vi "MAXI GAUGE - TREE.vi"   [LabVIEW 2013, in "Maxi Gauge.lvlib"]
uses:
  <instrlib>/Maxi Gauge/Maxi Gauge.lvlib
panel:
  # "SEE DIAGRAM FOR VI TREE"
  # "Pfeiffer Vacuum GmbH\n Berlinerstrasse 43\n D-35614 Asslar\n\n Telefon +49-6441/802-0\n Telefax +49-6441/802-202\n Internet: http://www.pfeiffer-vacuum.de"
  # "Maxi Gauge"
  # "07.01.2001 FPF"
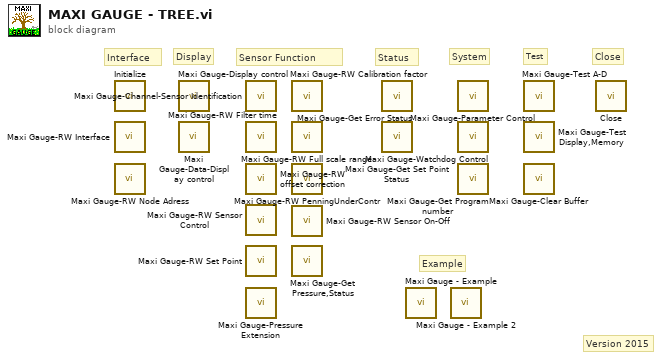
[diagram p0: block diagram]
diagram:
  # "Example"
  # "Close"
  # "Version 2015"
  # "Test"
  # "System"
  # "Status"
  # "Sensor Function"
  # "Display"
  # "Interface"
  n1 = call <instrlib>:"Initialize.vi"() -> ()  [unwired: 10 in, 2 out]
  n2 = call <instrlib>:"Maxi Gauge-RW Interface.vi"() -> ()  [unwired: 9 in, 3 out]
  n3 = call <instrlib>:"Maxi Gauge-RW Node Adress.vi"() -> ()  [unwired: 9 in, 3 out]
  n4 = call <instrlib>:"Maxi Gauge-Display control.vi"() -> ()  [unwired: 12 in, 4 out]
  n5 = call <instrlib>:"Maxi Gauge-Data-Display control.vi"() -> ()  [unwired: 11 in, 5 out]
  n6 = call <instrlib>:"Maxi Gauge-Channel-Sensor Identification.vi"() -> ()  [unwired: 8 in, 4 out]
  n7 = call <instrlib>:"Maxi Gauge-RW Filter time.vi"() -> ()  [unwired: 12 in, 8 out]
  n8 = call <instrlib>:"Maxi Gauge-RW offset correction.vi"() -> ()  [unwired: 12 in, 8 out]
  n9 = call <instrlib>:"Maxi Gauge-RW Sensor Control.vi"() -> ()  [unwired: 14 in, 6 out]
  n10 = call <instrlib>:"Maxi Gauge-RW Set Point.vi"() -> ()  [unwired: 11 in, 5 out]
  n11 = call <instrlib>:"Maxi Gauge-Pressure Extension.vi"() -> ()  [unwired: 12 in, 8 out]
  n12 = call <instrlib>:"Maxi Gauge-RW Calibration factor.vi"() -> ()  [unwired: 13 in, 3 out]
  n13 = call <instrlib>:"Maxi Gauge-RW Full scale range.vi"() -> ()  [unwired: 12 in, 8 out]
  n14 = call <instrlib>:"Maxi Gauge-RW PenningUnderContr.vi"() -> ()  [unwired: 12 in, 8 out]
  n15 = call <instrlib>:"Maxi Gauge-RW Sensor On-Off.vi"() -> ()  [unwired: 12 in, 8 out]
  n16 = call <instrlib>:"Maxi Gauge-Get Pressure,Status.vi"() -> ()  [unwired: 8 in, 4 out]
  n17 = call <instrlib>:"Maxi Gauge-Get Error Status.vi"() -> ()  [unwired: 7 in, 5 out]
  n18 = call <instrlib>:"Maxi Gauge-Get Set Point Status.vi"() -> ()  [unwired: 12 in, 8 out]
  n19 = call <instrlib>:"Maxi Gauge - Example.vi"() -> ()  [unwired: 9 in, 3 out]
  n20 = call <instrlib>:"Maxi Gauge - Example 2.vi"() -> ()  [unwired: 9 in, 3 out]
  n21 = call <instrlib>:"Maxi Gauge-Parameter Control.vi"() -> ()  [unwired: 9 in, 3 out]
  n22 = call <instrlib>:"Maxi Gauge-Watchdog Control.vi"() -> ()  [unwired: 9 in, 3 out]
  n23 = call <instrlib>:"Maxi Gauge-Get Program number.vi"() -> ()  [unwired: 9 in, 3 out]
  n24 = call <instrlib>:"Maxi Gauge-Test A-D.vi"() -> ()  [unwired: 12 in, 8 out]
  n25 = call <instrlib>:"Maxi Gauge-Test Display,Memory.vi"() -> ()  [unwired: 7 in, 5 out]
  n26 = call <instrlib>:"Maxi Gauge-Clear Buffer.vi"() -> ()  [unwired: 10 in, 2 out]
  n27 = call <instrlib>:"Close.vi"() -> ()  [unwired: 11 in, 1 out]
